vi "Type Color.vi"(11 "BooleanPanel in":refnum<class "BooleanPanel.lvclass">) -> (2 "Type Color":u32(colorbox))   [LabVIEW 2020, in "Conditum-Tools.lvlib" / "BooleanPanel.lvclass"]
uses:
  BooleanPanel.lvclass
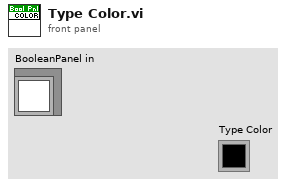
[diagram p1: front panel]
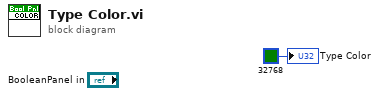
[diagram p0: block diagram]
diagram:
  "Type Color" <- u32 32768 ("Type Color")
